vi "GageAcquLoop.vi"(5 "GageParams.":T1={"Mode"=0, "Depth"=1024.0, "Segments"=1024, "Channel"=0} {"Mode" items=["Normal (0)"=0, "HWAverage (2)"=2, "MultiRecord (16)"=16]}, 7 "Refs.":T2, 8 "error in":errorcluster, 9 "SignalBufferQueue in":refnum<queue>, 11 "DWFCtrlQueue in":refnum<queue>) -> (0 "error out":errorcluster)   [LabVIEW 2013]
uses:
  Gage_States.ctl
  <instrlib>/GageLv_uic/Gage.lvlib
  ControlDef/Signal.ctl
  ControlDef/QuitProg.vi
  InstruGloble.vi
  ProcessMethods/SignalAverager/ProcessStates.ctl
  ProcessMethods/SignalAverager/DAQParams.ctl
  <instrlib>/ESP300/Public/Position_ESP300.vi
  <instrlib>/ESP300/ESP300.lvlib
  <instrlib>/Micos_uic/Public/Position_Micos.vi
  <instrlib>/Micos_uic/Micos_uic.lvlib
  <instrlib>/AnalogDiscSDKLv/VIs/DWF_Signal.ctl
  <instrlib>/AnalogDiscSDKLv/AnalogDiscSDKLv.lvlib
  GageAcqu.Refs.ctl
  GageParams.ctl
  <instrlib>/AnalogDiscSDKLv/VIs/DWF_State.ctl
  <instrlib>/AnalogDiscSDKLv/VIs/DWF_CtrlQueue.ctl
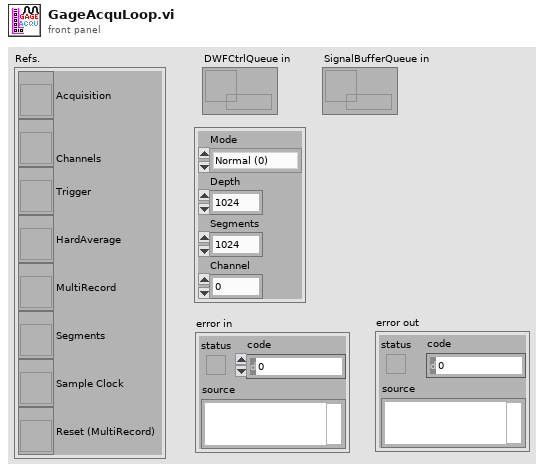
[diagram p1: front panel]
types:
  T1 = typedef "GageParams.ctl" = cluster{"Mode":u16, "Depth":dbl, "Segments":u32, "Channel":u16}
  T2 = typedef "GageAcqu.Refs.ctl" = cluster{"Acquisition":refnum<vi>, "Channels":refnum<vi>, "Trigger":refnum<vi>, "HardAverage":refnum<vi>, "MultiRecord":refnum<vi>, "Segments":refnum<vi>, "Sample Clock":refnum<vi>, "Reset (MultiRecord)":refnum<vi>}
  T3 = typedef "Gage_States.ctl" = enum16{"Initialize", "Config, Commit, Start", "Wait Idle", "Transfer", "CloseSystem"}
  T4 = cluster{"Handle":u32, "Sample size":u32, "Resolution":i32, "Offset":i32, "Channels":u32, "Boards":u32}
  T5 = typedef "Signal.ctl" = cluster{"Command":T6, "Params":variant}
  T6 = typedef "ProcessStates.ctl" = enum16{"Initialize", "Normal", "Display", "Write2Buffer", "CalcMzArray", "StartSave", "StopSave", "ConfigChanged", "EndOfLine", "SetFilterParams", "SetGraphsEnable", "SetAcquisitionParams", "ChangeDisplayIncrement", "ChangeRepRate", "SetWriterRef", "Quit", "StartOfLine"}
  T7 = typedef "DAQParams.ctl" = cluster{"TrigDelay":dbl, "Offset":i32, "Resolution":i32, "Range (mV)":u32, "Sample Rate":dbl, "Depth":dbl, "Segments":u32}
  T8 = typedef "AnalogDiscSDKLv.lvlib/DWF_Signal.ctl" = cluster{"tickcount":u32, "Signal":sgl[][], "SecondaryData":dbl[]}
  T9 = cluster{"Handle":u32, "Sample Size":u32, "Resolution":i32, "Offset":i32, "Channels":u32, "Boards":u32}
  T10 = typedef "AnalogDiscSDKLv.lvlib/DWF_CtrlQueue.ctl" = cluster{"DWF States":T11, "Variant":variant}
  T11 = typedef "AnalogDiscSDKLv.lvlib/DWF_State.ctl" = enum16{"Enumerate", "Open", "Close", "CloseAll", "Reset", "Quit", "==Settings==", "SetAcquisition_", "SetChannels_", "SetTrigger_", "SetAnalogTrigDetector_", "SetAll_AcquChTrig_", "fConfigurate", "fStart", "GetStatus", "_WaitForDone/Idle", "_GetData", "GetAcquisition", "GetChannels", "GetTrigger", "GetAll_AcquChTrig", "==Messaging==", "_PushDataOut", "GetStat_", "GetConfig_", "==ModeSetup==", "SetSignalBuffer_", "SetMode_", "SetSecondaryDataRef._", "==AnalogOut==", "GetChannelCount_AO", "fStart_AO", "SetChEnable_AO", "SetConfig_AO", "SetFuncData_AO", "SetOffset_AO_", "SetMasterNode_AO", "SetStates_AO", "SetSymetry_AO", "SetTriggerSource_AO", "==Trigger==", "ManualTrigger"}
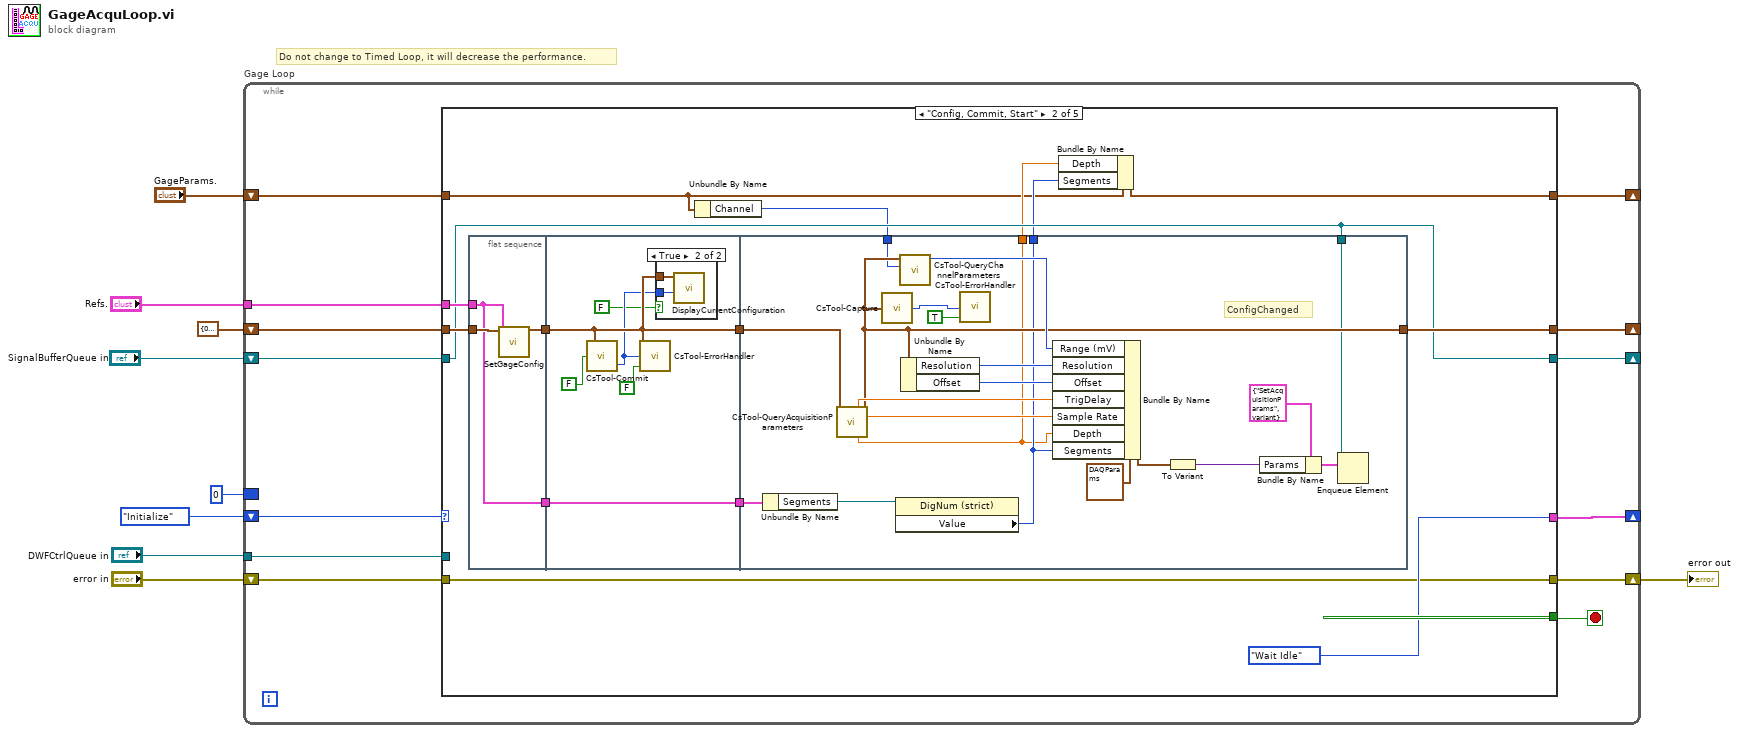
[diagram p0: block diagram]
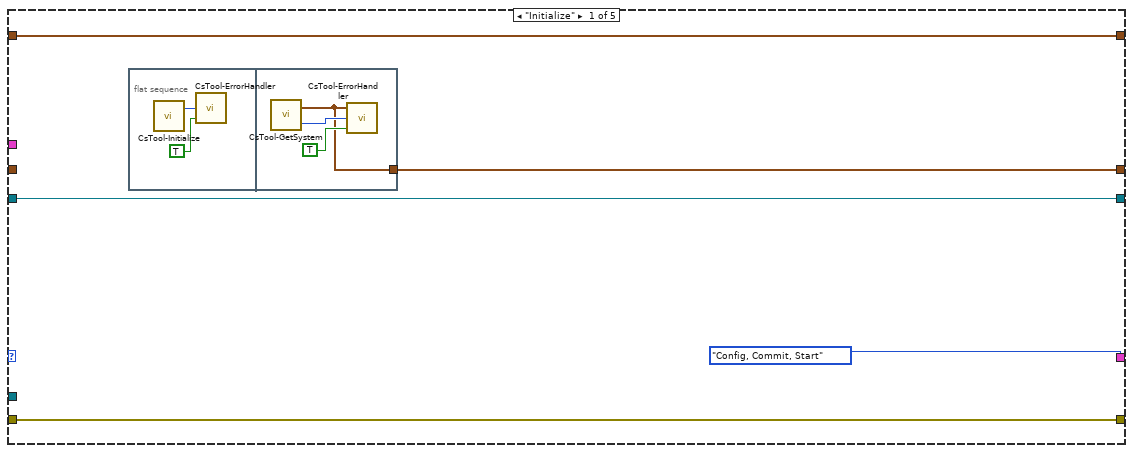
[diagram p2: hidden frame]
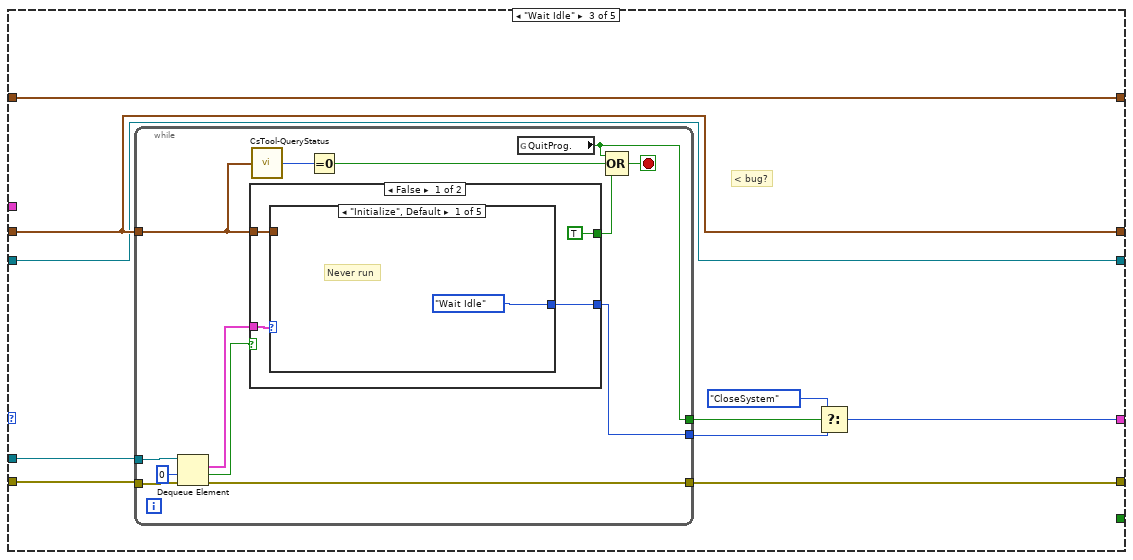
[diagram p4: hidden frame]
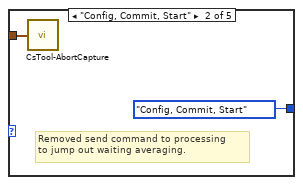
[diagram p5: hidden frame]
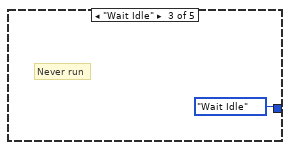
[diagram p6: hidden frame]
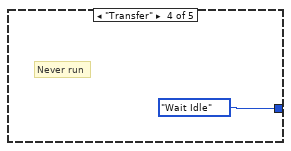
[diagram p7: hidden frame]
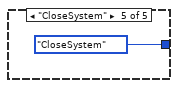
[diagram p8: hidden frame]
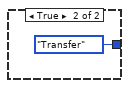
[diagram p9: hidden frame]
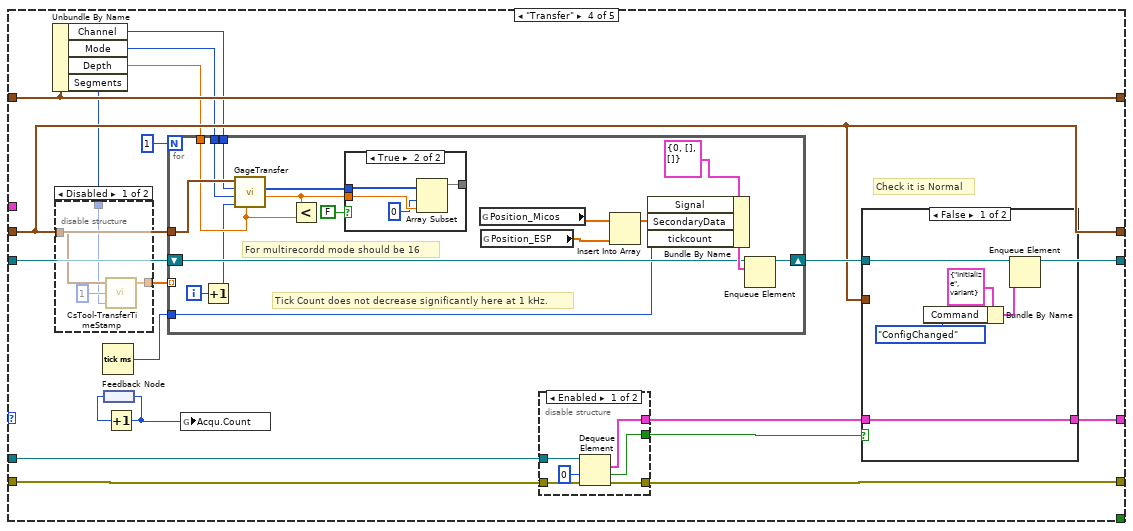
[diagram p10: hidden frame]
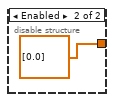
[diagram p11: hidden frame]
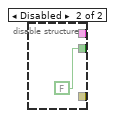
[diagram p13: hidden frame]
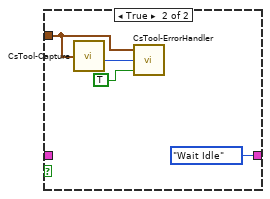
[diagram p14: hidden frame]
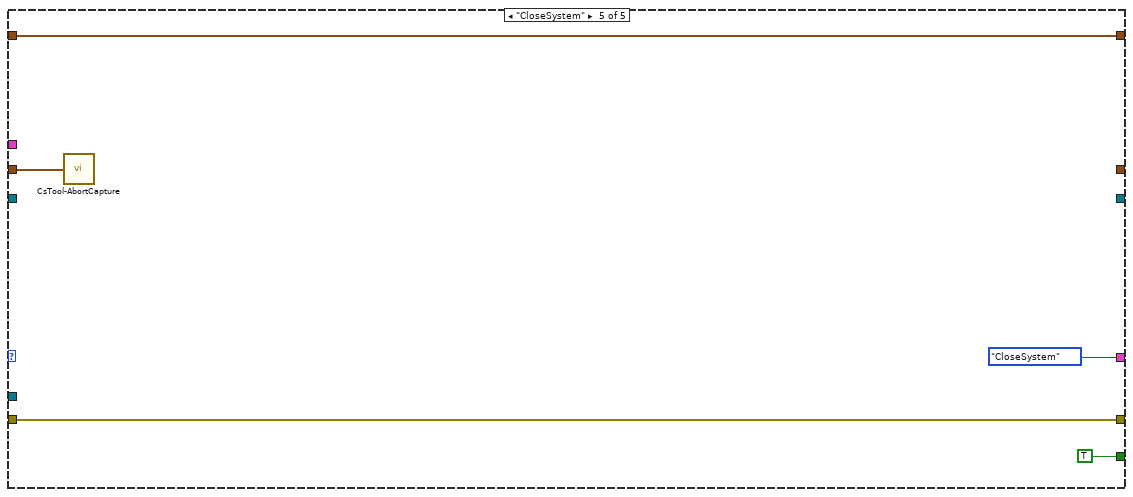
[diagram p15: hidden frame]
diagram:
  # "Do not change to Timed Loop, it will decrease the performance."
  n1 = while "Gage Loop" {
    shift-right: [w21] -> _
    shift-left: Gage_States."Initialize" ("Gage States") -> [w10]
    shift-right: [w20] -> _
    shift-left: "SignalBufferQueue in" -> [w22]
    shift-right: [w18] -> _
    shift-left: T4 {"Handle"=0, "Sample size"=0, "Resolution"=0, "Offset"=0, "Channels"=0, "Boards"=0} ("Handle Cluster") -> [w19]
    border: u32 0 ("Numeric") -> [_]
    tunnel: "DWFCtrlQueue in" -> [w16]
    shift-right: [w14] -> w3
    shift-left: "error in" -> [w15]
    tunnel: "Refs." -> [w13]
    shift-right: [w12] -> _
    shift-left: "GageParams." -> [w11]
    stop <- w17 stop-if-true
    n2 = case shown="\"Config, Commit, Start\"" w10 {
      tunnel: w22 -> [w26 w40 w83 w130 _]
      tunnel: [Gage_States."Config, Commit, Start" ("DAQ Status") Gage_States."Wait Idle" ("DAQ Status") w82 w124 Gage_States."CloseSystem" ("DAQ Status")] -> w21
      tunnel: [w26 w40 w83 w129 _] -> w20
      tunnel: w19 -> [_ w45 w87 w128 w177]
      tunnel: [w25 w44 w87 w128 _] -> w18
      tunnel: [_ _ _ _ TRUE] -> w17
      tunnel: w16 -> [_ _ w86 w127 _]
      tunnel: w15 -> [w24 w46 w85 w126 w174]
      tunnel: [w24 w46 w84 w125 w174] -> w14
      tunnel: w13 -> [_ w41 _ _ _]
      tunnel: [w23 w37 w79 w123 w175] -> w12
      tunnel: w11 -> [w23 w34 w79 w123 w175]
      frame "Initialize" {
        n3 = flat-sequence {
          tunnel: [w30] -> w25
          frame #0 {
            n4 = call <instrlib>:"CsTool-Initialize.vi"() -> ("Number Of Systems"=w29:i32)  [unwired: 1 out]
            n5 = call <instrlib>:"CsTool-ErrorHandler.vi"("StopOnError (true)"=TRUE, "Error Code"=w29) -> ()  [unwired: 1 in, 1 out]
          }
          frame #1 {
            n6 = call <instrlib>:"CsTool-GetSystem.vi"() -> ("Error Code"=w32:i32, "Handle Cluster"=w30:T4)  [unwired: 4 in]
            n7 = call <instrlib>:"CsTool-ErrorHandler.vi"("StopOnError (true)"=TRUE, "Error Code"=w32, "Handle Cluster"=w30) -> ()  [unwired: 1 out]
          }
        }
      }
      frame "Config, Commit, Start" {
        n8 = flat-sequence {
          tunnel: w45 -> [w49]
          tunnel: [w49] -> w43
          tunnel: w41 -> [w48]
          tunnel: [w48] -> w39
          tunnel: w43 -> [w53]
          tunnel: [w53] -> w42
          tunnel: w39 -> [w50]
          tunnel: [w50] -> w38
          tunnel: w42 -> [w75]
          tunnel: [w71] -> w44
          tunnel: w40 -> [w66]
          tunnel: w38 -> [w62]
          tunnel: [w60] -> w36
          tunnel: [w59] -> w35
          tunnel: w33 -> [w58]
          frame #0 {
            n9 = call "SetGageConfig.vi"("Gage Acqu."=w48, "Handle Cluster"=w49) -> ()  [unwired: 10 in]
          }
          frame #1 {
            n10 = call <instrlib>:"CsTool-Commit.vi"("Coerce Flag (f)"=FALSE, "Handle Cluster"=w53) -> ("Error Code"=w52:i32)  [unwired: 1 in, 1 out]
            n11 = call <instrlib>:"CsTool-ErrorHandler.vi"("StopOnError (true)"=FALSE, "Error Code"=w52, "Handle Cluster"=w53) -> ()  [unwired: 1 out]
            n12 = case shown="True" FALSE {
              tunnel: w53 -> [_ w57]
              tunnel: w52 -> [_ w56]
              frame False {
              }
              frame True {
                n13 = call <instrlib>:"DisplayCurrentConfiguration.vi"("error code  in"=w56, "Handle Cluster"=w57) -> ()  [unwired: 10 in]
              }
            }
          }
          frame #2 {
            # "ConfigChanged"
            n14 = Unbundle By Name(w62) -> ("Segments"=w61:refnum<vi>)
            n15 = call <instrlib>:"CsTool-QueryAcquisitionParameters.vi"("Handle Cluster"=w75) -> ("Trigger Delay"=w73:dbl, "Output Handle Cluster"=w71:T9, "Sample Rate"=w72:dbl, "Depth"=w59:dbl)  [unwired: 4 in, 7 out]
            n16 = call <instrlib>:"CsTool-Capture.vi"("Handle Cluster"=w71) -> ("Error Code"=w77:i32)
            n17 = property class="DigNum (strict)"(reference=w61) -> ("Value"=w60:u32)  [unwired: 1 in, 2 out]
            n18 = call <instrlib>:"CsTool-QueryChannelParameters.vi"("Handle Cluster"=w71, "Channel"=w58) -> ("Range (mV)"=w74:u32)  [unwired: 7 out]
            n19 = Unbundle By Name(w71) -> ("Resolution"=w70:i32, "Offset"=w69:i32)
            n20 = call <instrlib>:"CsTool-ErrorHandler.vi"("StopOnError (true)"=TRUE, "Error Code"=w77) -> ()  [unwired: 1 in, 1 out]
            n21 = Bundle By Name(cluster=T7 {"TrigDelay"=0.0, "Offset"=0, "Resolution"=-32768, "Range (mV)"=0, "Sample Rate"=100000000.0, "Depth"=16384.0, "Segments"=1} ("Value"), "Range (mV)"=w74, "Resolution"=w70, "Offset"=w69, "TrigDelay"=w73, "Sample Rate"=w72, "Depth"=w59, "Segments"=w60) -> (w64:T7)
            n22 = To Variant(anything=w64) -> (Variant=w63:variant)
            n23 = Bundle By Name(cluster=T5 {"Command"=enum."SetAcquisitionParams", "Params"=variant} ("element"), "Params"=w63) -> (w65:T5)
            n24 = Enqueue Element(queue=w66, element=w65) -> ()  [unwired: 2 in, 3 out]
          }
        }
        n25 = Unbundle By Name(w34) -> ("Channel"=w33:u16)
        n26 = Bundle By Name(cluster=w34, "Depth"=w35, "Segments"=w36) -> (w37:T1)
      }
      frame "Wait Idle" {
        # "< bug?"
        n27 = while "To get highest repetive rate,change waiting time to 0." {
          tunnel: w87 -> [w90]
          tunnel: w86 -> [w96]
          tunnel: w85 -> [w95]
          tunnel: [w92] -> w84
          tunnel: [w91] -> w81
          tunnel: [w88] -> w78
          stop <- w98 stop-if-true
          n28 = Dequeue Element(queue=w96, timeout in ms (-1)=0, error in (no error)=w95) -> (element=w94:T10, timed out?=w93:bool, error out=w92:errorcluster)  [unwired: 1 out]
          n29 = case shown="False" w93 {
            tunnel: [TRUE _] -> w97
            tunnel: w94 -> [w104 _]
            tunnel: [w103 Gage_States."Transfer" ("DAQ Status 2")] -> w91
            tunnel: w90 -> [w101 _]
            frame False {
              n30 = case shown="\"Initialize\", Default" w104 {
                tunnel: [Gage_States."Wait Idle" ("t") Gage_States."Config, Commit, Start" ("t") Gage_States."Wait Idle" ("t") Gage_States."Wait Idle" ("t") Gage_States."CloseSystem" ("t")] -> w103
                tunnel: w101 -> [_ w106 _ _ _]
                frame "Initialize", Default {
                  # "Never run"
                }
                frame "Config, Commit, Start" {
                  # "Removed send command to processing\nto jump out waiting averaging."
                  n31 = call <instrlib>:"CsTool-AbortCapture.vi"("Handle Cluster"=w106) -> ()  [unwired: 1 out]
                }
                frame "Wait Idle" {
                  # "Never run"
                }
                frame "Transfer" {
                  # "Never run"
                }
                frame "CloseSystem" {
                }
              }
            }
            frame True {
            }
          }
          n32 = call <instrlib>:"CsTool-QueryStatus.vi"("Handle Cluster"=w90) -> ("Status"=w100:i32)
          n33 = Equal To 0?(x=w100) -> (x = 0?=w99:bool)
          n34 = global read "QuitProg.vi" "QuitProg."() -> (w88:bool)
          n35 = Compound Arithmetic op=OR(w88, w99, w97) -> (w98:bool)
        }
        n36 = Select(t=Gage_States."CloseSystem", s=w78, f=w81) -> (s? t:f=w82:T3)
      }
      frame "Transfer" {
        # "Check it is Normal"
        n37 = Unbundle By Name(w123) -> ("Channel"=w115:u16, "Mode"=w114:u16, "Depth"=w122:dbl, "Segments"=w116:u32)
        n38 = disable-structure shown="Disabled" {
          disable-tunnel: w128 -> [w134 _]
          disable-tunnel: [w132 dbl[] [0.0]] -> w117
          disable-tunnel: w116 -> [w131 _]
          frame Disabled {
            n39 = call <instrlib>:"CsTool-TransferTimeStamp.vi"("Length (1)"=w131, "Segment (1)"=u32 1, "Handle Cluster"=w134) -> ("TS Time"=w132:dbl[])  [unwired: 2 out]
          }
          frame Enabled {
          }
        }
        n40 = Tick Count (ms)() -> (millisecond timer value=w113:u32)
        n41 = feedback #1() -> (w121:u32)
        n42 = Increment(x=w121) -> (x+1=w120:u32)
        n43 = feedback-in #1(w120) -> ()
        n44 = for {
          N: 1 -> [_]
          tunnel: w128 -> [w151]
          tunnel: w122 -> [w148]
          shift-right: [w152] -> w129
          shift-left: w130 -> [w146]
          tunnel: w117 -> [_] mode=indexing
          tunnel: w115 -> [w143]
          tunnel: w114 -> [w142]
          tunnel: w113 -> [w141]
          i -> [w145]
          # "For multirecordd mode should be 16"
          # "Tick Count does not decrease significantly here at 1 kHz."
          n45 = Increment(x=w145) -> (x+1=w144:i32)
          n46 = call "GageTransfer.vi"("Length (4096)"=w148, "Segment (1)"=w144, "Mode (0)"=w142, "Channel (0)"=w143, "Handle Cluster"=w151) -> ("Actual Length"=w149:dbl, "Data_Raw"=w150:i32[])  [unwired: 3 in, 2 out]
          n47 = Less?(x=w149, y=w148) -> ()  [unwired: 1 out]
          n48 = case shown="True" FALSE {
            tunnel: w150 -> [w153 w157]
            tunnel: [w153 w154] -> _
            tunnel: w149 -> [_ w156]
            frame False {
            }
            frame True {
              n49 = Array Subset(array=w157, index=0, length=w156) -> (w154:i32[])
            }
          }
          n50 = global read "Position_Micos.vi" "Position_Micos"() -> (w137:dbl[])
          n51 = global read "Position_ESP300.vi" "Position_ESP"() -> (w139:dbl[])
          n52 = Insert Into Array(array=w137, new element=w139) -> (w138:dbl[])  [unwired: 1 in]
          n53 = Bundle By Name(cluster=T8 {"tickcount"=0, "Signal"=[], "SecondaryData"=[]} ("Signal_Typedef"), "SecondaryData"=w138, "tickcount"=w141) -> (w147:T8)  [unwired: 1 in]
          n54 = Enqueue Element(queue=w146, element=w147) -> (queue out=w152:refnum<queue>)  [unwired: 2 in, 2 out]
        }
        n55 = global write "InstruGloble.vi" "Acqu.Count"(w120) -> ()
        n56 = disable-structure shown="Enabled" {
          disable-tunnel: w127 -> [w163 _]
          disable-tunnel: w126 -> [w162 _]
          disable-tunnel: [w161 _] -> w125
          disable-tunnel: [w160 FALSE ("timed out?")] -> w119
          disable-tunnel: [w159 _] -> w118
          frame Enabled {
            n57 = Dequeue Element(queue=w163, timeout in ms (-1)=0, error in (no error)=w162) -> (element=w159:T10, timed out?=w160:bool, error out=w161:errorcluster)  [unwired: 1 out]
          }
          frame Disabled {
          }
        }
        n58 = case shown="False" w119 {
          tunnel: w128 -> [_ w171]
          tunnel: w118 -> [w169 _]
          tunnel: [w169 Gage_States."Wait Idle" ("Gage States")] -> w124
          tunnel: w129 -> [w167 _]
          frame False {
            n59 = Bundle By Name(cluster=T5 {"Command"=enum."Initialize", "Params"=variant} ("element"), "Command"=ProcessStates."ConfigChanged") -> (w166:T5)
            n60 = Enqueue Element(queue=w167, element=w166) -> ()  [unwired: 2 in, 3 out]
          }
          frame True {
            n61 = call <instrlib>:"CsTool-Capture.vi"("Handle Cluster"=w171) -> ("Error Code"=w173:i32)
            n62 = call <instrlib>:"CsTool-ErrorHandler.vi"("StopOnError (true)"=TRUE, "Error Code"=w173, "Handle Cluster"=w171) -> ()  [unwired: 1 out]
          }
        }
      }
      frame "CloseSystem" {
        n63 = call <instrlib>:"CsTool-AbortCapture.vi"("Handle Cluster"=w177) -> ()  [unwired: 1 out]
      }
    }
  }
  "error out" <- w3
